vi "GEA2 Serial Find Valid Com Ports.vi"(0 "Valid Com Port List(100,2:56)":u8[](array[numeric])) -> (4 "Valid Com Ports":refnum<visa-resource-name>[](array[refnum]), 6 "Found?":bool)   [LabVIEW 2014]
uses:
  <vilib>/Instr/_visa.llb/VISA Find Search Mode.ctl
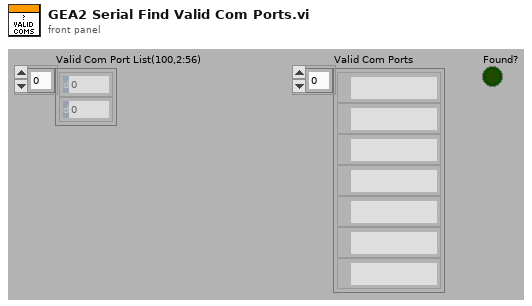
[diagram p1: front panel]
types:
  T1 = typedef "VISA Find Search Mode.ctl" = u32
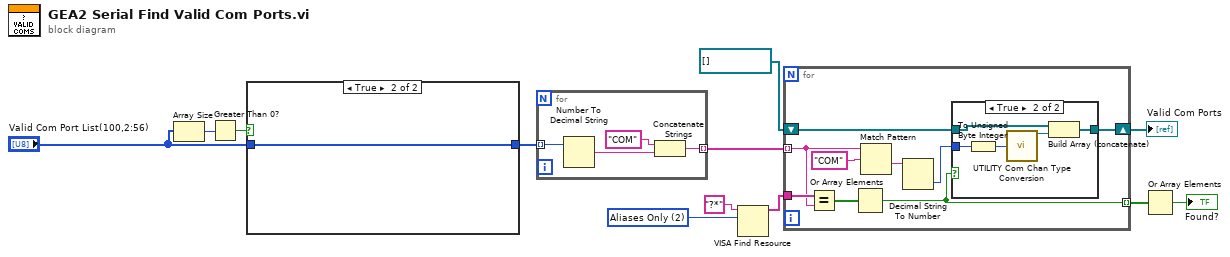
[diagram p0: block diagram]
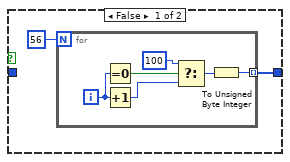
[diagram p2: hidden frame]
diagram:
  w12 = T1 2 items=["Canonical Names Only"=0, "Aliases Only"=2, "Include Matching Aliases"=3, "Include All Aliases"=4] ("Search Mode")
  n1 = Array Size(array="Valid Com Port List(100,2:56)") -> (size(s)=w7:i32)
  n2 = Greater Than 0?(x=w7) -> (x > 0?=w8:bool)
  n3 = case shown="True" w8 {
    tunnel: [w13 w21] -> w6
    tunnel: "Valid Com Port List(100,2:56)" -> [_ w21]
    frame False {
      n4 = for {
        N: 56 -> [_]
        tunnel: [w15] -> w13 mode=indexing
        i -> [w20]
        n5 = Equal To 0?(x=w20) -> (x = 0?=w18:bool)
        n6 = Increment(x=w20) -> (x+1=w19:i32)
        n7 = Select(t=100, s=w18, f=w19) -> (s? t:f=w16:i32)
        n8 = To Unsigned Byte Integer(number=w16) -> (unsigned 8bit integer=w15:u8)
      }
    }
    frame True {
    }
  }
  n9 = for {
    tunnel: [w23] -> w1 mode=indexing
    tunnel: w6 -> [w22] mode=indexing
    n10 = Number To Decimal String(number=w22) -> (decimal integer string=w25:string)  [unwired: 1 in]
    n11 = Concatenate Strings("COM", w25) -> (w23:string)
  }
  n12 = VISA Find Resource(10:w12, 11:"?*" ("expression (\"?*\")")) -> (3:w2:string[])  [unwired: 1 in, 2 out]
  n13 = for {
    tunnel: w1 -> [w30] mode=indexing
    tunnel: w2 -> [w34]
    shift-right: [w32] -> w9
    shift-left: refnum<visa-resource-name>[] [] -> [w31]
    tunnel: [w26] -> w4 mode=indexing
    n14 = Equal?(x=w34, y=w30) -> (x = y?=w33:bool[])
    n15 = Or Array Elements(Boolean array=w33) -> (logical OR=w26:bool)
    n16 = Match Pattern(string=w30, regular expression="COM") -> (after substring=w28:string)  [unwired: 1 in, 3 out]
    n17 = Decimal String To Number(string=w28) -> (number=w27:i32)  [unwired: 2 in, 1 out]
    n18 = case shown="True" w26 {
      tunnel: [w35 w40] -> w32
      tunnel: w31 -> [w35 w38]
      tunnel: w27 -> [_ w37]
      frame False {
      }
      frame True {
        n19 = To Unsigned Byte Integer(number=w37) -> (unsigned 8bit integer=w36:u8)
        n20 = call "UTILITY Com Chan Type Conversion.vi"("Com Chan"=w36) -> ("VISA resource name"=w39:refnum<visa-resource-name>)  [unwired: 11 in, 3 out]
        n21 = Build Array (concatenate)(w38, w39) -> (w40:refnum<visa-resource-name>[])
      }
    }
  }
  "Valid Com Ports" <- w9
  n22 = Or Array Elements(Boolean array=w4) -> (logical OR=→"Found?":bool)
